vi "Configure Transient Trigger Source.vi"(8 "error in (no error)":errorcluster, 10 "Transient Trigger Source (0: Bus)":u16(ring) items=["Bus", "External", "Immediate", "Pin 1", "Pin 2", "Pin 3", "Pin 4", "Pin 5", "Pin 6", "Pin 7"], 11 "VISA resource name":refnum<visa-resource-name>) -> (0 "error out":errorcluster, 3 "VISA resource name out":refnum<visa-resource-name>)   [LabVIEW 2021, in "Agilent N6900 N7900 Series.lvlib"]
doc: "Selects the trigger source for the transient system."
uses:
  <instrlib>/Agilent N6900 N7900 Series/Agilent N6900 N7900 Series.lvlib
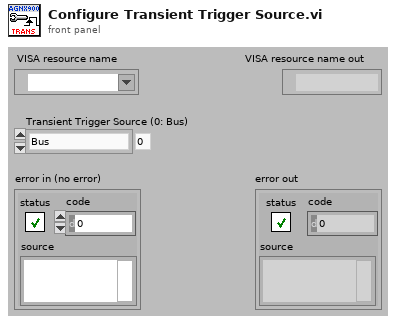
[diagram p1: front panel]
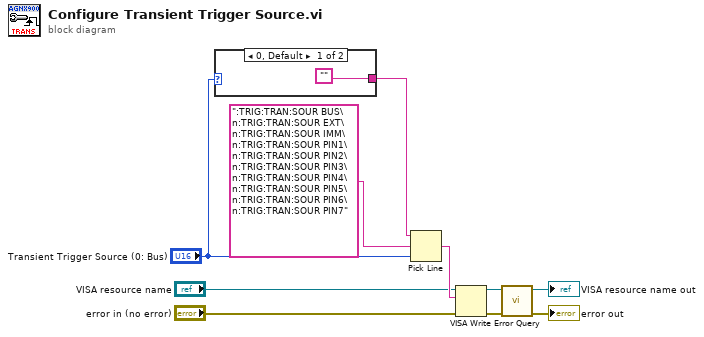
[diagram p0: block diagram]
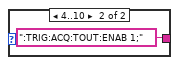
[diagram p2: hidden frame]
diagram:
  n1 = case shown="0, Default" "Transient Trigger Source (0: Bus)" {
    tunnel: ["" ("string (\"\")") ":TRIG:ACQ:TOUT:ENAB 1;" ("string (\"\")")] -> w8
    frame 0, Default {
    }
    frame 4..10 {
    }
  }
  n2 = Pick Line(string ("")=w8, multi-line string=":TRIG:TRAN:SOUR BUS\n:TRIG:TRAN:SOUR EXT\n:TRIG:TRAN:SOUR IMM\n:TRIG:TRAN:SOUR PIN1\n:TRIG:TRAN:SOUR PIN2\n:TRIG:TRAN:SOUR PIN3\n:TRIG:TRAN:SOUR PIN4\n:TRIG:TRAN:SOUR PIN5\n:TRIG:TRAN:SOUR PIN6\n:TRIG:TRAN:SOUR PIN7", line index="Transient Trigger Source (0: Bus)") -> (output string=w3:string)
  n3 = VISA Write(VISA resource name="VISA resource name", write buffer=w3, error in (no error)="error in (no error)") -> (VISA resource name out=w4:refnum<visa-resource-name>, error out=w5:errorcluster)  [unwired: 1 out]
  n4 = call <instrlib>:"Error Query.vi"("error in (no error)"=w5, "VISA resource name"=w4) -> ("error out"=→"error out":errorcluster, "VISA resource name out"=→"VISA resource name out":refnum<visa-resource-name>)  [unwired: 6 in, 2 out]
